vi "Open Connection.vi"(8 "error in (no error)":errorcluster, 10 "IP":string, 11 "Network Stream in":refnum<class "Network Stream.lvclass">) -> (0 "error out":errorcluster, 3 "Network Stream out":refnum<class "Network Stream.lvclass">)   [LabVIEW 2019, in "Network Stream.lvlib" / "Network Stream.lvclass"]
uses:
  Network Stream.lvclass
  C:/Program Files (x86)/National Instruments/LabVIEW 2019/vi.lib/ActorFramework/Actor/Actor.lvclass
  Network Stream.lvclass/Network Stream.ctl
  <vilib>/ActorFramework/Actor/Actor.lvclass/Actor.ctl
  Network Stream Messages/NS Connection Msg/NS Connection Msg.lvclass/NS Connection Msg.ctl
  <vilib>/ActorFramework/Message Enqueuer/Message Enqueuer.lvclass/Message Enqueuer.ctl
  <vilib>/ActorFramework/Message Enqueuer/Enqueue.vi
  Network Stream Messages/NS Connection Msg/NS Connection Msg.lvclass
  C:/Program Files (x86)/National Instruments/LabVIEW 2019/vi.lib/ActorFramework/Message/Message.lvclass
  <vilib>/ActorFramework/Message Priority Queue/Priority Enqueue.vi
  <resource>/objmgr/ni.dex.rc
  <vilib>/ActorFramework/Actor/Actor.lvclass
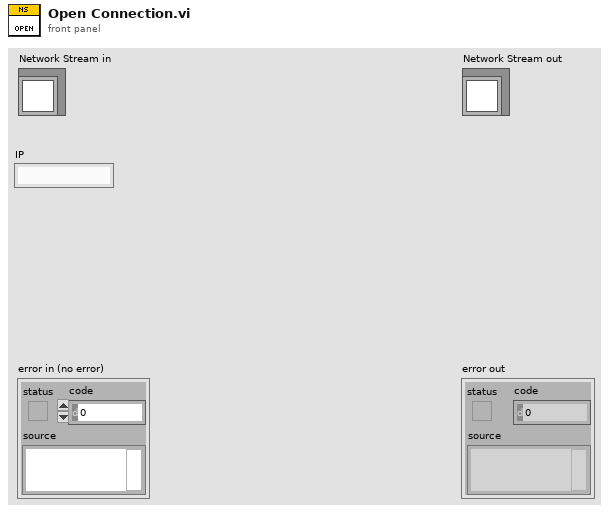
[diagram p1: front panel]
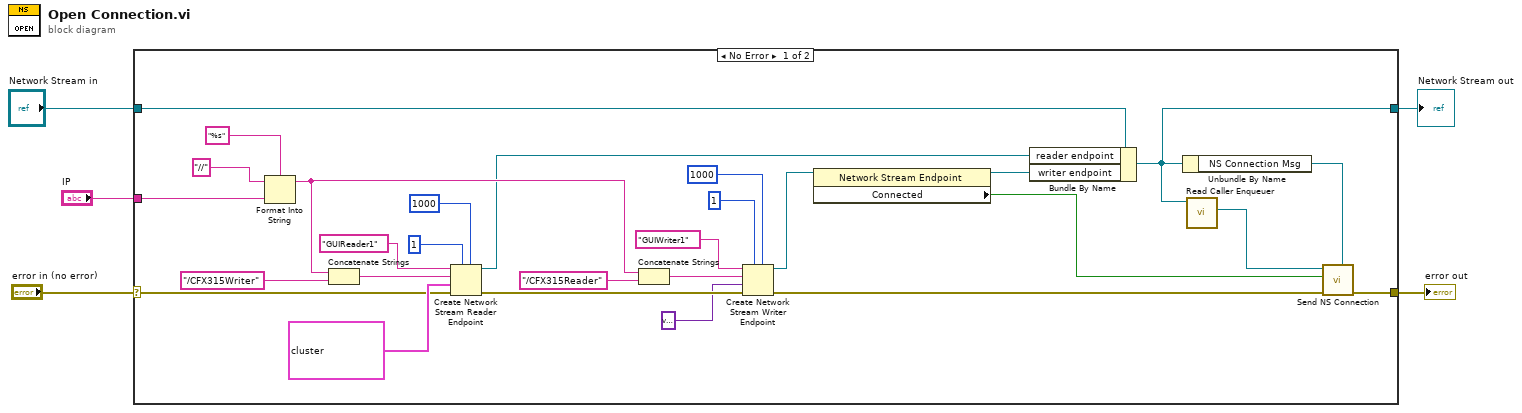
[diagram p0: block diagram]
diagram:
  n1 = case shown="No Error" "error in (no error)" {
    selector: "error in (no error)" -> [w17 w35]
    tunnel: [w9 w35] -> w4
    tunnel: [w11 w34] -> w2
    tunnel: "Network Stream in" -> [w15 w34]
    tunnel: "IP" -> [w16 _]
    frame No Error {
      n2 = Format Into String(format string="%s", initial string="//" ("string"), w16) -> (resulting string=w33:string)  [unwired: 1 in, 1 out]
      n3 = Concatenate Strings(w33, "/CFX315Writer" ("string")) -> (w23:string)
      n4 = Create Network Stream Reader Endpoint(5:1000 ("timeout in ms (-1)"), 7:1 ("reader buffer size"), 8:w17, 9:cluster{"Data":variant, "Timestamp":timestamp} {"Data"=variant, "Timestamp"=timestamp(0 s since 1904-01-01)} ("Dataset"), 10:w23, 11:"GUIReader1" ("reader name")) -> (0:w29:errorcluster, 3:w14:refnum<k21>)  [unwired: 1 in]
      n5 = Concatenate Strings(w33, "/CFX315Reader" ("writer name")) -> (w28:string)
      n6 = Create Network Stream Writer Endpoint(5:1000 ("timeout in ms (-1)"), 7:1 ("writer buffer size"), 8:w29, 9:variant, 10:w28, 11:"GUIWriter1" ("writer name")) -> (0:w10:errorcluster, 3:w13:refnum<k21>)  [unwired: 1 in]
      n7 = property class="Network Stream Endpoint"(reference=w13) -> (reference out=w12:refnum<k21>, "Connected"=w6:bool)  [unwired: 1 in, 1 out]
      n8 = Bundle By Name(cluster=w15, "reader endpoint"=w14, "writer endpoint"=w12) -> (w11:refnum<class "Network Stream.lvclass">)
      n9 = Unbundle By Name(w11) -> ("NS Connection Msg"=w7:refnum<class "NS Connection Msg.lvclass">)
      n10 = call <vilib>:"Read Caller Enqueuer.vi"("Actor"=w11) -> ("Caller Enqueuer"=w8:refnum<class "Message Enqueuer.lvclass">)  [unwired: 10 in]
      n11 = call "Send NS Connection.vi"("Message Type"=w7, "error in (no error)"=w10, "NS Conn"=w6, "Message Enqueuer"=w8) -> ("error out"=w9:errorcluster)  [unwired: 6 in, 1 out]
    }
    frame Error {
    }
  }
  "error out" <- w4
  "Network Stream out" <- w2
